vi "SwerveLatchGoalAngle.vi"(1 "Raw Goal Angle":dbl format="%#_13g", 2 "In Deadband":bool) -> (0 "Latched Goal Angle":dbl)   [LabVIEW 2019]
doc: "Latches the goal azimuth angle when the driver releases the stick. This prevents the modules from slewing to a new orientation and jerking the robot."
uses:
  sensors.vi
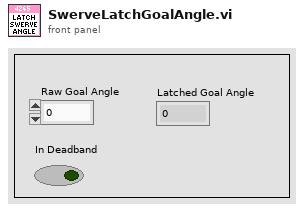
[diagram p1: front panel]
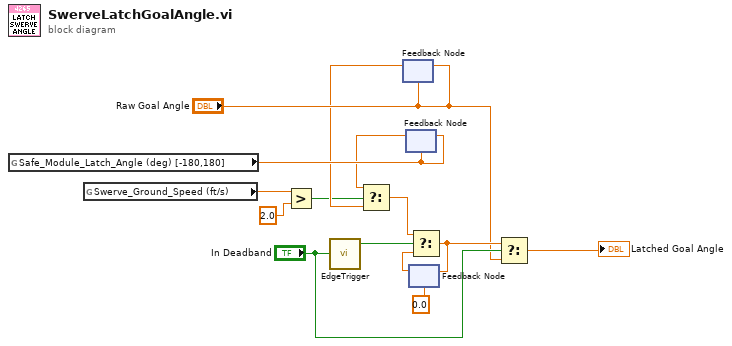
[diagram p0: block diagram]
diagram:
  n1 = global read "sensors.vi" "Safe_Module_Latch_Angle (deg) [-180,180]"() -> (w8:dbl)
  n2 = global read "sensors.vi" "Swerve_Ground_Speed (ft/s)"() -> (w3:dbl)
  n3 = Greater?(x=w3, y=2.0) -> (0:w2:bool)
  n4 = call "EdgeTrigger.vi"("Input Signal"="In Deadband") -> ("Rising Edge Trigger"=w14:bool)  [unwired: 2 out]
  n5 = feedback-in #1("Raw Goal Angle") -> ()
  n6 = feedback #1("Raw Goal Angle") -> (w5:dbl)
  n7 = feedback-in #2(w8) -> ()
  n8 = feedback #2(w8) -> (w4:dbl)
  n9 = Select(t=w4, s=w2, f=w5) -> (s? t:f=w6:dbl)
  n10 = feedback #3(0.0) -> (w12:dbl)
  n11 = Select(t=w6, s=w14, f=w12) -> (s? t:f=w11:dbl)
  n12 = feedback-in #3(w11) -> ()
  n13 = Select(t=w11, s="In Deadband", f="Raw Goal Angle") -> (s? t:f=→"Latched Goal Angle":dbl)
